vi "save config.vi"(8 "error in (no error)":errorcluster, 10 "file config":string, 11 "Channel in":refnum<class "Channel.lvclass">) -> (0 "error out":errorcluster, 3 "Channel out":refnum<class "Channel.lvclass">)   [LabVIEW 2018, in "Channel.lvclass"]
uses:
  Channel.lvclass
  Channel.lvclass/Channel.ctl
  <vilib>/Utility/config.llb/Write Key (String).vi
  <vilib>/Utility/config.llb/NI_LVConfig.lvlib
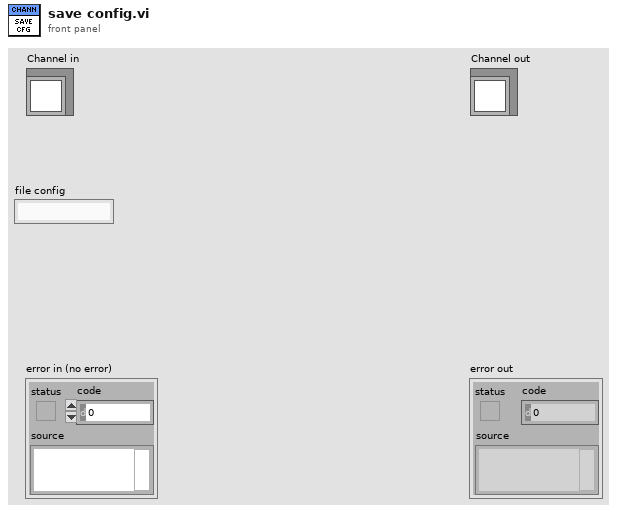
[diagram p1: front panel]
types:
  T1 = cluster{"ACQUISITION_MODE":u8, "TRIGGER_MODE":u8, "READ_MODE":u8, "PREAMP":u8, "READOUT_RATE":u8, "VERTICAL_SHIFT_SPEED":u8, "EM_MODE":u8, "EM_GAIN":u16, "SHUTTER_MODE":u8, "SHUTTER_TTL":u8, "SHUTTER_OPENING_TIME":u16, "SHUTTER_CLOSING_TIME":u16, "VBIN":u16, "HBIN":u16, "INITIAL_LINE":u16, "INITIAL_COLUMN":u16, "FINAL_LINE":u16, "FINAL_COLUMN":u16, "FRAME_TRANSFER":bool, "VERTICAL_CLOCK_VOLTAGE":u8, "AD_CHANNEL":u32}
  T2 = typedef "NI_LVConfig.lvlib/Config Data RefNum.ctl" = refnum<k1>
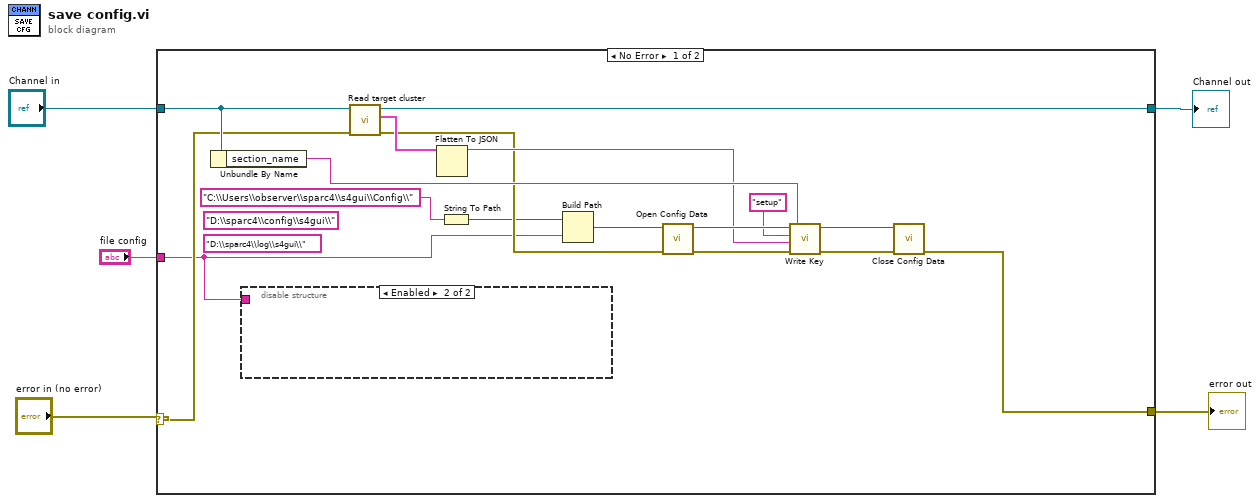
[diagram p0: block diagram]
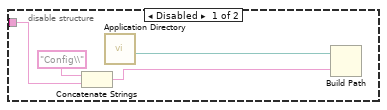
[diagram p2: hidden frame]
diagram:
  n1 = case shown="No Error" "error in (no error)" {
    selector: "error in (no error)" -> [w10 w28]
    tunnel: [w14 w28] -> w2
    tunnel: [w11 w27] -> w3
    tunnel: "Channel in" -> [w13 w27]
    tunnel: "file config" -> [w7 _]
    frame No Error {
      (unwired) "D:\\sparc4\\log\\s4gui\\" ("default name")
      (unwired) "D:\\sparc4\\config\\s4gui\\" ("default name")
      n2 = Unbundle By Name(w13) -> ("section_name"=w21:string)
      n3 = disable-structure shown="Enabled" {
        disable-tunnel: w7 -> [w24 _]
        frame Disabled {
          n4 = Concatenate Strings("Config\\" ("key"), w24) -> (w23:string)
          n5 = call <vilib>:"Application Directory.vi"() -> ("Application Directory"=w26:path)
          n6 = Build Path(base path=w26, name or relative path=w23) -> ()  [unwired: 1 out]
        }
        frame Enabled {
        }
      }
      n7 = call-dynamic "Read target cluster.vi"("error in (no error)"=w10, "Channel in"=w13) -> ("error out"=w9:errorcluster, "target cluster"=w12:T1, "Channel out"=w11:refnum<class "Channel.lvclass">)  [unwired: 7 in]
      n8 = Flatten To JSON(anything=w12) -> (JSON string=w15:string)  [unwired: 2 in, 1 out]
      n9 = String To Path(string="C:\\Users\\observer\\sparc4\\s4gui\\Config\\") -> (path=w8:path)
      n10 = Build Path(base path=w8, name or relative path=w7) -> (appended path=w22:path)
      n11 = call <vilib>:"Open Config Data.vi"("error in (no error)"=w9, "configuration file path"=w22) -> ("error out"=w18:errorcluster, "refnum"=w20:T2)  [unwired: 7 in, 1 out]
      n12 = call-poly <vilib>:"Write Key.vi"("section"=w21, "error in (no error)"=w18, "value"=w15, "key"="setup", "refnum"=w20) -> ("error out"=w16:errorcluster, "refnum out"=w17:T2)  [unwired: 4 in, 1 out]
      n13 = call <vilib>:"Close Config Data.vi"("error in (no error)"=w16, "refnum"=w17) -> ("error out"=w14:errorcluster)  [unwired: 8 in, 1 out]
    }
    frame Error {
    }
  }
  "error out" <- w2
  "Channel out" <- w3
